vi "Create (EAST).vi"(5 "Non-Maximum Suppression (Default: 0.0)":sgl, 7 "Confidence Threshold (Default: 0.5)":sgl=0.5, 8 "error in (no error)":errorcluster, 11 "Model":T1) -> (0 "error out":errorcluster, 3 "Text Detector":refnum<class "Text Detector.lvclass">)   [LabVIEW 2020, in "feature_detection.lvlib" / "Text Detector.lvclass"]
doc: "Create a DNN based DB type Text Detector. See for more details https://docs.opencv.org/4.11.0/db/d0f/classcv_1_1dnn_1_1TextDetectionModel__DB.html"
uses:
  Text Detector.lvclass
  Text Detector.lvclass/Text Detector.ctl
  common/common.lvlib
  common/bin/gartoolkit_dnn_32-1.dll
  common/Image Size (Integer).ctl
  common/Object Point (Float).ctl
  Model.ctl
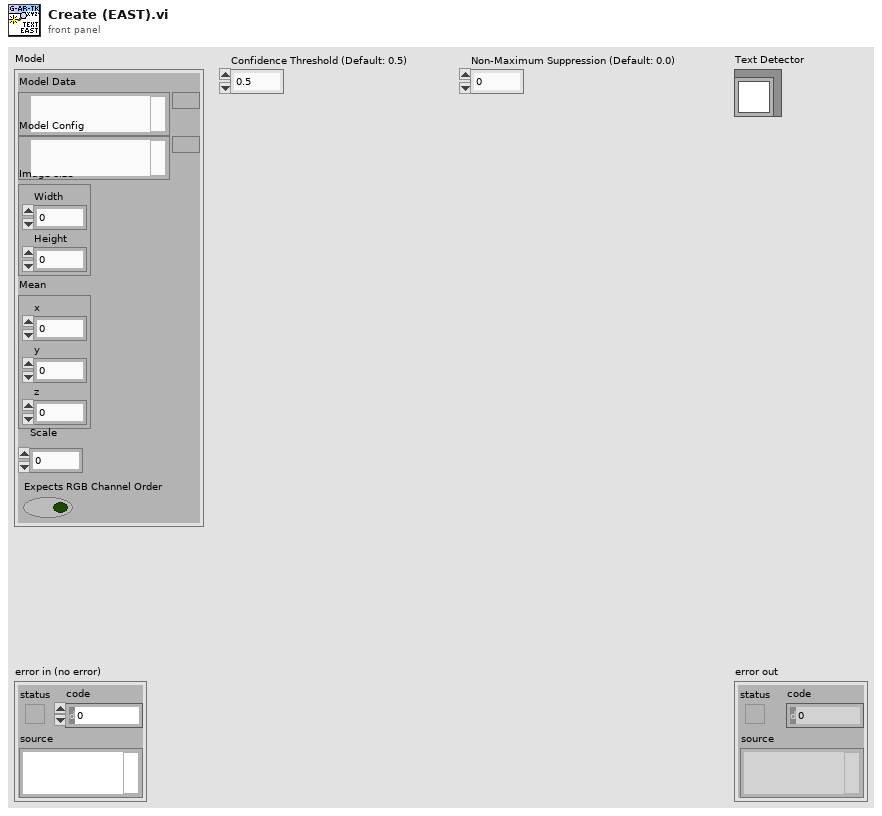
[diagram p1: front panel]
types:
  T1 = typedef "feature_detection.lvlib/Text Detector.lvclass/Model.ctl" = cluster{"Model Data":path, "Model Config":path, "Image Size":T2, "Mean":T3, "Scale":dbl, "Expects RGB Channel Order":bool}
  T2 = typedef "common.lvlib/Image Size (Integer).ctl" = cluster{"Width":u16, "Height":u16}
  T3 = typedef "common.lvlib/Object Point (Float).ctl" = cluster{"x":dbl, "y":dbl, "z":dbl}
  T4 = cluster{"Model Data":string, "Model Config":string, "Image Size":T2, "Mean":T3, "Scale":dbl, "Expects RGB Channel Order":bool}
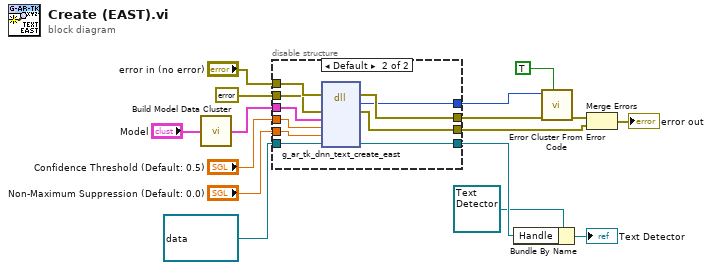
[diagram p0: block diagram]
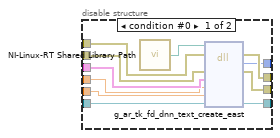
[diagram p2: hidden frame]
diagram:
  n1 = call "Build Model Data Cluster.vi"("Model in"="Model") -> ("Model out"=w1:T4)
  n2 = disable-structure "Conditional Disable Structure" shown="Default" {
    disable-tunnel: "error in (no error)" -> [w26 w37]
    disable-tunnel: errorcluster {"status"=FALSE, "code"=0, "source"=""} ("error constant") -> [w27 w36]
    disable-tunnel: refnum<data-value> refnum ("EDVR") -> [w22 w35]
    disable-tunnel: [w20 w34] -> w13
    disable-tunnel: [w19 w33] -> w12
    disable-tunnel: [w18 w32] -> w11
    disable-tunnel: [w17 w31] -> w10
    disable-tunnel: w1 -> [w25 w30]
    disable-tunnel: "Confidence Threshold (Default: 0.5)" -> [w24 w29]
    disable-tunnel: "Non-Maximum Suppression (Default: 0.0)" -> [w23 w28]
    frame condition #0 {
      n3 = call "NI-Linux-RT Shared Library Path.vi"() -> ("Path"=w21:path)
      n4 = dll-call lib="?" fn="g_ar_tk_fd_dnn_text_create_east" ("g_ar_toolkit.*.*:g_ar_tk_capture_context_create")(path in=w21, error in=w26, "error_cluster"=w27, "model"=w25, "conf_threshold"=w24, "nms_threshold"=w23, "EDVR"=w22) -> (error out=w20:errorcluster, "return type"=w19:i32, "error_cluster"=w17:errorcluster, "EDVR"=w18:refnum<data-value>)  [unwired: 4 in, 1 out]
    }
    frame condition #1 (active) {
      n5 = dll-call lib="C:/serenial/lib/g-augmented-reality-toolkit/LabVIEW/common/bin/gartoolkit_dnn_*-1.*" fn="g_ar_tk_dnn_text_create_east" ("g_ar_toolkit.*.*:g_ar_tk_capture_context_create")(error in=w37, "error_cluster"=w36, "model"=w30, "conf_threshold"=w29, "nms_threshold"=w28, "EDVR"=w35) -> (error out=w34:errorcluster, "return type"=w33:i32, "error_cluster"=w31:errorcluster, "EDVR"=w32:refnum<data-value>)  [unwired: 5 in, 1 out]
    }
  }
  n6 = Bundle By Name(cluster=refnum<class "Text Detector.lvclass"> refnum ("Text Detector in"), "Handle"=w11) -> (→"Text Detector":refnum<class "Text Detector.lvclass">)
  n7 = call <vilib>:"Error Cluster From Error Code.vi"("show call chain? (False)"=TRUE, "error in (no error)"=w13, "error code (0)"=w12) -> ("error out"=w16:errorcluster)  [unwired: 6 in]
  n8 = Merge Errors(w16, w10) -> (→"error out":errorcluster)
